vi "Sub_SetNormalPara.vi"(0 "Iset":u32, 1 "Imax":u32, 2 "Channel":i32, 3 "Device Handle":u32) -> ()   [LabVIEW 2013]
uses:
  x64_lib/Mightex_LEDDriver_SDK.dll
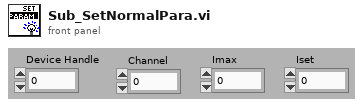
[diagram p1: front panel]
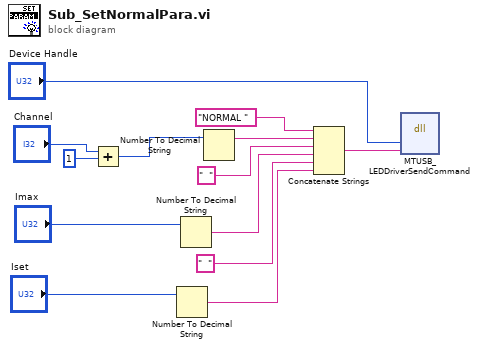
[diagram p0: block diagram]
diagram:
  n1 = Add(x="Channel", y=1) -> (x+y=w1:i32)
  n2 = Number To Decimal String(number="Iset") -> (decimal integer string=w9:string)  [unwired: 1 in]
  n3 = Number To Decimal String(number="Imax") -> (decimal integer string=w11:string)  [unwired: 1 in]
  n4 = Number To Decimal String(number=w1) -> (decimal integer string=w5:string)  [unwired: 1 in]
  n5 = Concatenate Strings("NORMAL ", w5, "  ", w11, "  ", w9) -> (w12:string)
  n6 = dll-call lib="C:/Users/ignacio/Desktop/Patrick's File Reader Function/led_control/documentation/SDK/x64_lib/Mightex_LEDDriver_SDK.dll" fn="MTUSB_LEDDriverSendCommand"("arg1"="Device Handle", "arg2"=w12) -> ()  [unwired: 6 in, 2 out]
